vi "LVClass_WavefrontCorrector get Parameter Values SetAndGet.vi"(0 "WavefrontCorrector in":refnum<class "WavefrontCorrector.lvclass">, 11 "error in (no error)":errorcluster) -> (4 "WavefrontCorrector out":refnum<class "WavefrontCorrector.lvclass">, 6 "ListOfSettableAndGettableValue":T1[](array[typedef]), 15 "error out":errorcluster)   [LabVIEW 2020, in "WavefrontCorrector.lvclass"]
doc: "Description:\nGet current actuators positions.\n\nParameters:\nclass corrector WavefrontCorrector object adress.\nfloat position Array containing the actuators positions.\nError error_in [in] Error\nError error_out [out] Error"
uses:
  WavefrontCorrector.lvclass
  Controls/CameraParametersSetup.ctl
  Controls/CameraParameters_Type.ctl
  WavefrontCorrector.lvclass/WavefrontCorrector.ctl
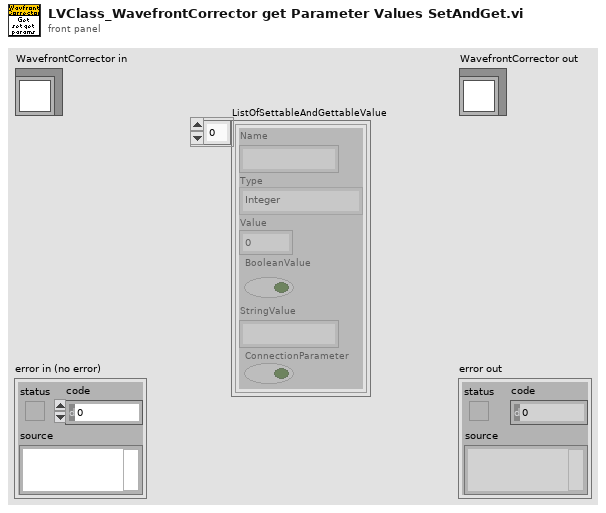
[diagram p1: front panel]
types:
  T1 = typedef "CameraParametersSetup.ctl" = cluster{"Name":string, "Type":T2, "Value":dbl, "BooleanValue":bool, "StringValue":string, "ConnectionParameter":bool}
  T2 = typedef "CameraParameters_Type.ctl" = enum16{"Integer", "Real", "String", "Boolean"}
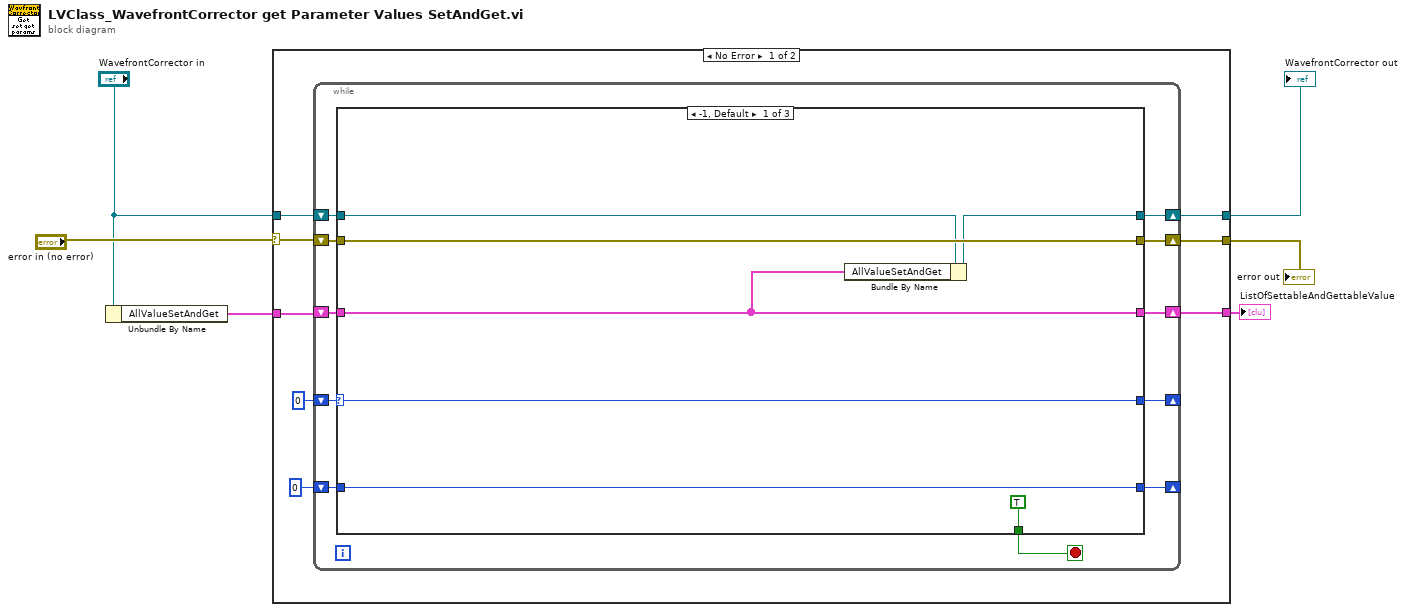
[diagram p0: block diagram]
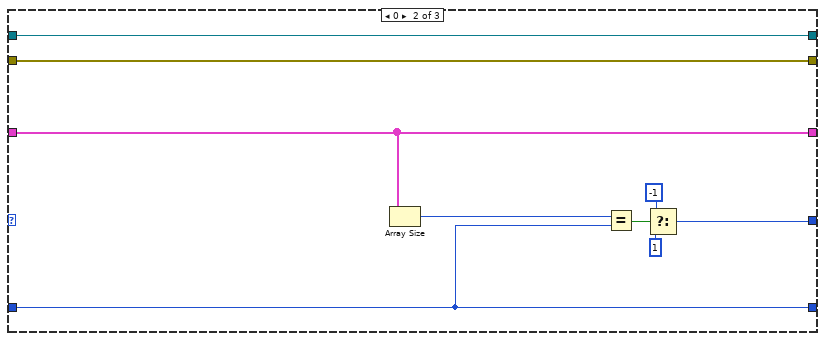
[diagram p2: hidden frame]
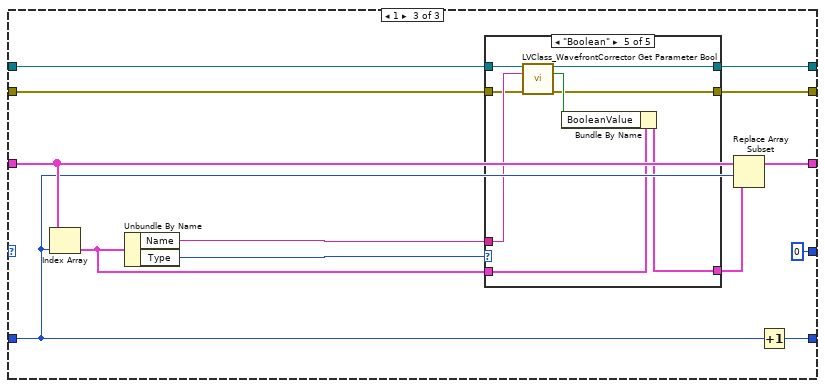
[diagram p3: hidden frame]
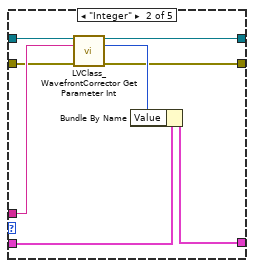
[diagram p5: hidden frame]
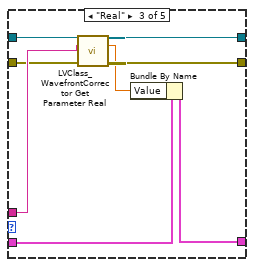
[diagram p6: hidden frame]
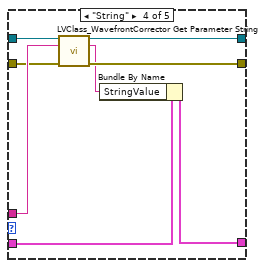
[diagram p7: hidden frame]
diagram:
  n1 = Unbundle By Name("WavefrontCorrector in") -> ("AllValueSetAndGet"=w1:T1[])
  n2 = case shown="No Error" "error in (no error)" {
    selector: "error in (no error)" -> [w10 w91]
    tunnel: [w11 w91] -> w4
    tunnel: [w12 w90] -> w6
    tunnel: "WavefrontCorrector in" -> [w14 w90]
    tunnel: [w9 _] -> w3
    tunnel: w1 -> [w7 _]
    frame No Error {
      n3 = while {
        shift-right: [w24] -> _
        shift-left: 0 -> [w23]
        shift-right: [w21] -> w11
        shift-left: w10 -> [w20]
        shift-right: [w22] -> w12
        shift-left: w14 -> [w25]
        shift-right: [w18] -> w9
        shift-left: w7 -> [w17]
        shift-right: [w15] -> _
        shift-left: 0 -> [w16]
        stop <- w19 stop-if-true
        n4 = case shown="-1, Default" w23 {
          selector: w23 -> [w29 _ _]
          tunnel: w25 -> [w28 w41 w42]
          tunnel: w20 -> [w31 w40 w43]
          tunnel: [w29 w34 0] -> w24
          tunnel: [w27 w41 w53] -> w22
          tunnel: [w31 w40 w52] -> w21
          tunnel: [TRUE _ _] -> w19
          tunnel: [w26 w39 w47] -> w18
          tunnel: w17 -> [w26 w39 w49]
          tunnel: w16 -> [w30 w37 w48]
          tunnel: [w30 w37 w51] -> w15
          frame -1, Default {
            n5 = Bundle By Name(cluster=w28, "AllValueSetAndGet"=w26) -> (w27:refnum<class "WavefrontCorrector.lvclass">)
          }
          frame 0 {
            n6 = Array Size(array=w39) -> (size(s)=w38:i32)
            n7 = Equal?(x=w38, y=w37) -> (x = y?=w36:bool)
            n8 = Select(t=-1, s=w36, f=1) -> (s? t:f=w34:i32)
          }
          frame 1 {
            n9 = Index Array(array=w49, index=w48) -> (element=w50:T1)
            n10 = Unbundle By Name(w50) -> ("Name"=w45:string, "Type"=w46:T2)
            n11 = case shown="\"Boolean\"" w46 {
              tunnel: w50 -> [w55 w65 w66 w74 w83]
              tunnel: [w55 w64 w67 w81 w82] -> w44
              tunnel: w45 -> [_ w63 w72 w78 w88]
              tunnel: w42 -> [w57 w62 w73 w80 w89]
              tunnel: [w57 w61 w69 w79 w86] -> w53
              tunnel: [w56 w59 w70 w76 w84] -> w52
              tunnel: w43 -> [w56 w58 w71 w77 w87]
              frame Default {
              }
              frame "Integer" {
                n12 = call "LVClass_WavefrontCorrector Get Parameter Int.vi"("WavefrontCorrector in"=w62, "parameter_name"=w63, "error in (no error)"=w58) -> ("WavefrontCorrector out"=w61:refnum<class "WavefrontCorrector.lvclass">, "value"=w60:i32, "error out"=w59:errorcluster)  [unwired: 10 in]
                n13 = Bundle By Name(cluster=w65, "Value"=w60) -> (w64:T1)
              }
              frame "Real" {
                n14 = call "LVClass_WavefrontCorrector Get Parameter Real.vi"("WavefrontCorrector in"=w73, "parameter_name"=w72, "error in (no error)"=w71) -> ("WavefrontCorrector out"=w69:refnum<class "WavefrontCorrector.lvclass">, "value"=w68:dbl, "error out"=w70:errorcluster)  [unwired: 10 in]
                n15 = Bundle By Name(cluster=w66, "Value"=w68) -> (w67:T1)
              }
              frame "String" {
                n16 = call "LVClass_WavefrontCorrector Get Parameter String.vi"("WavefrontCorrector in"=w80, "parameter_name"=w78, "error in (no error)"=w77) -> ("WavefrontCorrector out"=w79:refnum<class "WavefrontCorrector.lvclass">, "value"=w75:string, "error out"=w76:errorcluster)  [unwired: 10 in]
                n17 = Bundle By Name(cluster=w74, "StringValue"=w75) -> (w81:T1)
              }
              frame "Boolean" {
                n18 = call "LVClass_WavefrontCorrector Get Parameter Bool.vi"("WavefrontCorrector in"=w89, "parameter_name"=w88, "error in (no error)"=w87) -> ("WavefrontCorrector out"=w86:refnum<class "WavefrontCorrector.lvclass">, "value"=w85:bool, "error out"=w84:errorcluster)  [unwired: 10 in]
                n19 = Bundle By Name(cluster=w83, "BooleanValue"=w85) -> (w82:T1)
              }
            }
            n20 = Replace Array Subset(array=w49, new element=w44, index=w48) -> (w47:T1[])
            n21 = Increment(x=w48) -> (x+1=w51:i32)
          }
        }
      }
    }
    frame Error {
    }
  }
  "error out" <- w4
  "WavefrontCorrector out" <- w6
  "ListOfSettableAndGettableValue" <- w3
